vi "Sub_Read_Fixed_Header.vi"(8 "error in (no error)":errorcluster, 11 "SSL_Connection":T1) -> (0 "error out":errorcluster, 1 "MessageType":T2, 2 "Remaining Length":u32, 3 "SSL_Connection":T1, 5 "QoS Level":T3, 6 "DUP Flag":bool, 7 "RETAIN":bool)   [LabVIEW 2018, in "AWS_IoT.lvlib"]
uses:
  AWS_IoT.lvlib
  Controls/QoS.ctl
  Controls/MessageType.ctl
  Controls/SSL_Connection.ctl
panel:
  out "data out":u8[](array[numeric]) format="%x"
  # "fixed header"
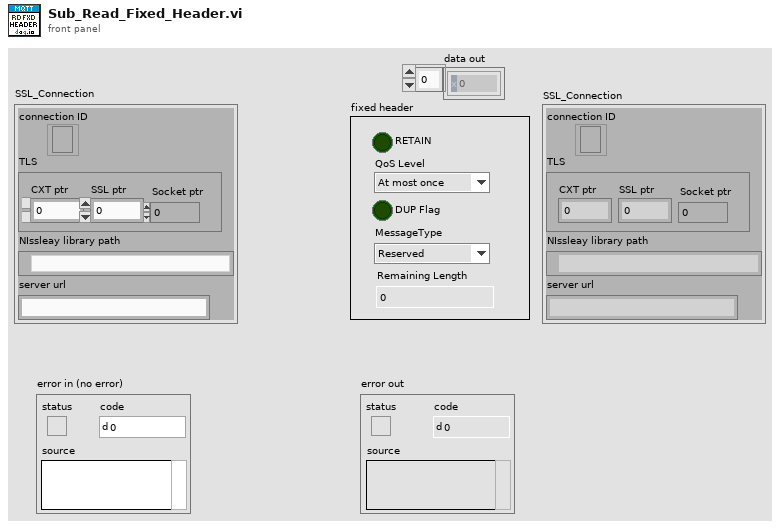
[diagram p1: front panel]
types:
  T1 = typedef "AWS_IoT.lvlib/SSL_Connection.ctl" = cluster{"connection ID":refnum<k5>, "TLS":cluster{"CXT ptr":i32, "SSL ptr":i32, "Socket ptr":i32}, "NIssleay library path":path, "server url":string}
  T2 = typedef "AWS_IoT.lvlib/MessageType.ctl" = enum32{"Reserved", "CONNECT", "CONNACK", "PUBLISH", "PUBACK", "PUBREC", "PUBREL", "PUBCOMP", "SUBSCRIBE", "SUBACK", "UNSUBSCRIBE", "UNSUBACK", "PINGREQ", "PINGRESP", "DISCONNECT", "Reserved2"}
  T3 = typedef "AWS_IoT.lvlib/QoS.ctl" = enum8{"At most once", "At least once", "Exactly once", "Reserved"}
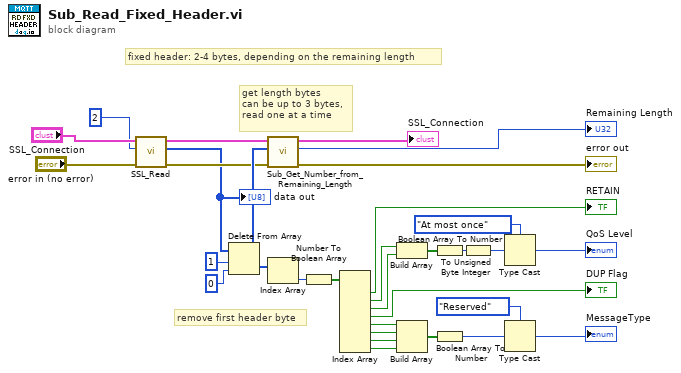
[diagram p0: block diagram]
diagram:
  # "fixed header: 2-4 bytes, depending on the remaining length"
  # "get length bytes\ncan be up to 3 bytes,\nread one at a time"
  # "remove first header byte"
  n1 = call "SSL_Read.vi"("error in (no error)"="error in (no error)", "bytes to read"=2, "SSL_Connection"="SSL_Connection") -> ("error out"=w8:errorcluster, "data out"=w3:u8[], "SSL_Connection"=w4:T1)  [unwired: 5 in, 1 out]
  "data out" <- w3
  n2 = Delete From Array(array=w3, length=1, index=0) -> (deleted portion=w28:u8[], array with subset deleted=w10:u8[])
  n3 = call "Sub_Get_Number_from_Remaining_Length.vi"("error in (no error)"=w8, "Remaining Length"=w10, "SSL_Connection"=w4) -> ("error out"=→"error out":errorcluster, "X"=→"Remaining Length":u32, "SSL_Connection"=→"SSL_Connection":T1)  [unwired: 6 in]
  n4 = Index Array(array=w28) -> (element=w27:u8)  [unwired: 1 in]
  n5 = Number To Boolean Array(number=w27) -> (Boolean array=w26:bool[])
  n6 = Index Array(array=w26) -> (element #1=→"RETAIN":bool, element #2=w24:bool, element #3=w23:bool, element #4=→"DUP Flag":bool, element #5=w19:bool, element #6=w18:bool, element #7=w17:bool, element #8=w16:bool)  [unwired: 8 in]
  n7 = Build Array(w24, w23) -> (w22:bool[])
  n8 = Build Array(w19, w18, w17, w16) -> (w15:bool[])
  n9 = Boolean Array To Number(Boolean array=w22) -> (number=w12:u32)
  n10 = Boolean Array To Number(Boolean array=w15) -> (number=w13:u32)
  n11 = To Unsigned Byte Integer(number=w12) -> (unsigned 8bit integer=w6:u8)
  n12 = Type Cast(type=QoS."At most once" ("QoS"), x=w6) -> (*(type *) &x=→"QoS Level":T3)
  n13 = Type Cast(type=MessageType."Reserved" ("MessageType"), x=w13) -> (*(type *) &x=→"MessageType":T2)
